vi "play_AFM_PI.vi"() -> ()   [LabVIEW 2017]
uses:
  controls/controlParams_tracktraj.ctl
  <vilib>/Analysis/Matrix/Datatypes/RealMatrix.ctl
  fpga_fp_interface_lib/fpga_interface_types/boolean_indicators.ctl
  <vilib>/userdefined/High Color/nirio_resource_hc.ctl
  <vilib>/Utility/error.llb/DialogType.ctl
  <vilib>/Utility/file.llb/Read From Spreadsheet File (DBL).vi
  <vilib>/FPGAPlugInAG/cRIO-9082/niLvFpga_Open_cRIO-9082.vi
  <vilib>/rvi/interface/common/dynamic/niFpgaDynamicAddResources.vi
  <vilib>/FPGAPlugInAG/Dynamic/niLvFpga_Reset_Dynamic.vi
  <vilib>/rvi/interface/common/niFpgaWaitOnOcc.vi
  <vilib>/Utility/error.llb/Error Cluster From Error Code.vi
  <vilib>/rvi/errors/niLvFpgaAdjustHostInterfaceError.vi
  <vilib>/FPGAPlugInAG/Dynamic/niLvFpga_Run_Dynamic.vi
  fpga_fp_interface_lib/write_FP_data_to_fpga.vi
  fpga_fp_interface_lib/acquire_fp_yk_FIFO.vi
  <vilib>/Utility/file.llb/Write To Spreadsheet File (DBL).vi
  <vilib>/Analysis/Matrix/Numeric/Conversions/Array To Matrix - RA2.vi
  <vilib>/FPGAPlugInAG/Dynamic/niLvFpga_Close_Dynamic.vi
  <vilib>/rvi/interface/nirviOpenFPGA/nirviOpenFPGA.xnode
  FPGA Bitfiles/XYpeizocontrol_FPGATargetSPARTA_AFM_PI_control.lvbitx
  <vilib>/rvi/interface/nirviMethod/nirviMethod.xnode
  <vilib>/rvi/interface/nirviReadWriteControl/nirviReadWriteControl.xnode
  <vilib>/rvi/interface/nirviCloseFPGA/nirviCloseFPGA.xnode
  <vilib>/FPGAPlugInAG/Dynamic/niLvFpga_ConfigureFifo_Dynamic.vi
  <vilib>/rvi/errors/niLvFpgaMergeErrorWithErrorCode.vi
  <vilib>/rvi/interface/Simulation/niFpgaSimulationCallBeginRW.vi
  <vilib>/Analysis/Matrix/NI_Matrix.lvlib
  <vilib>/FPGAPlugInAG/Dynamic/niLvFpga_WriteFifo_Dynamic.vi
  NiFpgaLv.dll
panel:
  in  "Tab Control":enum32{"MAIN", "Page 1", "Debug Info"}(tab)
  out "XY Graph":cluster{dbl[], "2D Data Out":dbl[]}[](graph)
  in  "traj_path":path=path "Z:/mpc-journal/step-exps/ref_traj_track.csv"
  in  "TsTicks":i32=1600
  in  "umax":dbl=1.0 format="%#_13g"
  in  "ymax":dbl=4.0 format="%#_13g"
  in  "Iters":i32=25
  in  "SettleTicks":i32=10
  in  "outputDataPath":path=path "Z:/mpc-journal/step-exps/expOut_multiAxis_tmp.csv"
  in  "Kp":sgl
  in  "Ki":dbl=0.125346917944 format="%#_13g"
  in  "ABORT":bool
  out "result_data":T1
  out "boolean  indicators":T2
  out "u_k out":fxp<+/-,32,5>
  out "size(s) 2":i32[](array[numeric])
  out "error out":errorcluster
  out "Actual Depth":u32
  out "error out 2":errorcluster
  out "elements left":i32=1
  in  "Cluster":T3={"umax"=3.0, "y_ref(k)"=0.0, "Ki"=0.0, "y(k) (from plant)"=0.0, "ND"=0, "NS"=0, "u_Kx_ref(k)"=0.0, "du_max"=3.0, "NS_obs"=0, "NS_control"=0, "Kp"=0.0} {"Kp" format="%#_13g"; "du_max" format="%#_13g"; "u_Kx_ref(k)" format="%#_13g"; "Ki" format="%#_13g"; "y_ref(k)" format="%#_13g"; "umax" format="%#_13g"}
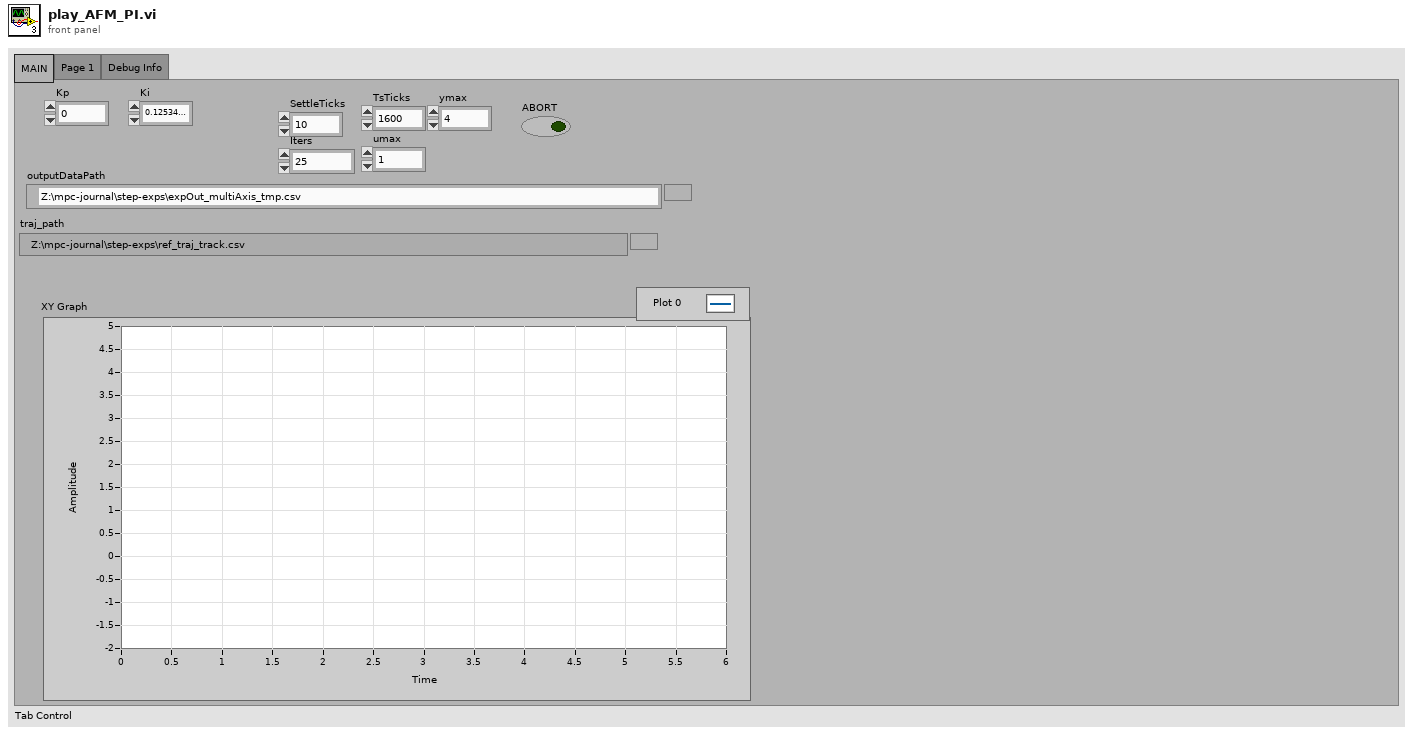
[diagram p1: front panel]
types:
  T1 = typedef "NI_Matrix.lvlib/RealMatrix.ctl" = dbl[][]
  T2 = typedef "boolean_indicators.ctl" = cluster{"unstable-z-traj":bool, "input fifo time-out":bool, "logging fifo timeout":bool, "scanning finished":bool, "unstable-x-traj":bool, "unstable-y-traj":bool, "ABORT":bool, "All Measurements Done":bool, "fpga_finished":bool}
  T3 = typedef "controlParams_tracktraj.ctl" = cluster{"umax":sgl, "y_ref(k)":sgl, "Ki":sgl, "y(k) (from plant)":sgl, "ND":i16, "NS":i16, "u_Kx_ref(k)":sgl, "du_max":sgl, "NS_obs":i16, "NS_control":i16, "Kp":sgl}
  T4 = typedef "nirio_resource_hc.ctl" = tag
  T5 = cluster{"unstable-z-traj":bool, "input fifo time-out":bool, "logging fifo timeout":bool, "scanning finished":bool, "unstable-x-traj":bool, "unstable-y-traj":bool, "ABORT":bool, "All Measurements Done":bool, "fpga_finished":bool}
  T6 = typedef "DialogType.ctl" = u16
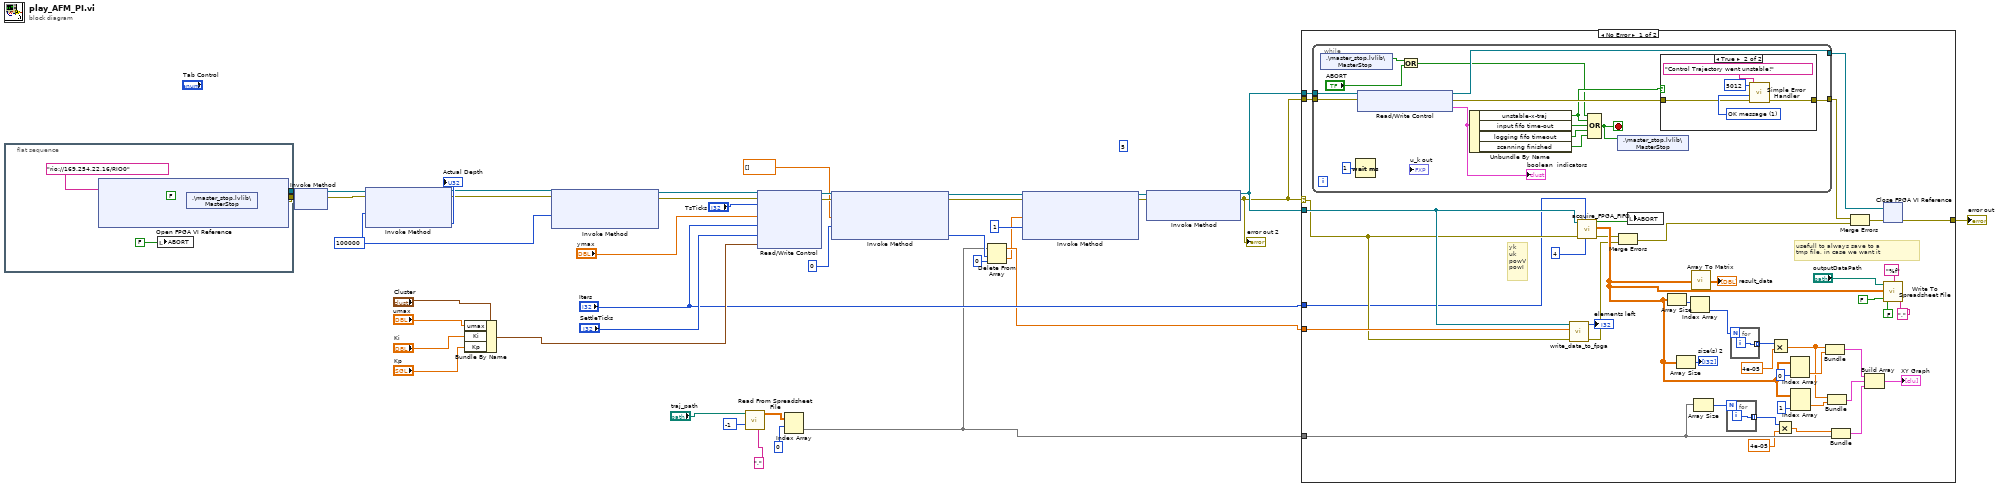
[diagram p0: block diagram]
diagram:
  (unwired) 5
  w34 = 100000
  n1 = flat-sequence {
    tunnel: [w47] -> w33
    tunnel: [w45] -> w4
    frame #0 {
      n2 = xnode "Open FPGA VI Reference"("resource name"=T4 "rio://169.254.22.16/RIO0") -> ("FPGA VI Reference Out"=w47:refnum<k20>, "error out"=w44:errorcluster)  [unwired: 1 in]
      n3 = local write "ABORT"(FALSE ("MasterStop")) -> ()
      n4 = shared-variable ".\\master_stop.lvlib\\MasterStop"(FALSE ("MasterStop"), error in=w44) -> (error out=w45:errorcluster)
    }
  }
  n5 = xnode "Invoke Method"("FPGA VI Reference In"=w33, "error in"=w4) -> ("FPGA VI Reference Out"=w39:refnum<k20>, "error out"=w38:errorcluster)
  n6 = xnode "Invoke Method"("FPGA VI Reference In"=w39, "error in"=w38, "Requested Depth"=w34) -> ("FPGA VI Reference Out"=w7:refnum<k20>, "error out"=w6:errorcluster, "Actual Depth"=→"Actual Depth":u32)
  n7 = Bundle By Name(cluster="Cluster", "umax"="umax", "Ki"="Ki", "Kp"="Kp") -> (w24:T3)
  n8 = xnode "Invoke Method"("FPGA VI Reference In"=w7, "error in"=w6, "Requested Depth"=w34) -> ("FPGA VI Reference Out"=w36:refnum<k20>, "error out"=w35:errorcluster)  [unwired: 1 out]
  n9 = call-poly <vilib>:"Read From Spreadsheet File.vi"("delimiter (\\t)"=",", "number of rows (all:-1)"=-1, "file path (dialog if empty)"="traj_path") -> ("all rows"=w28:dbl[][])  [unwired: 4 in, 4 out]
  n10 = xnode "Read/Write Control"("FPGA VI Reference In"=w36, "error in"=w35, "TsTicks"="TsTicks", "ymax"="ymax", "iters"="Iters", "Settle Ticks"="SettleTicks", "ControlParms"=w24) -> ("FPGA VI Reference Out"=w20:refnum<k20>, "error out"=w19:errorcluster)
  n11 = Index Array(array=w28, index (row)=0 ("dimension size")) -> (element=w1:dbl[])  [unwired: 1 in]
  n12 = xnode "Invoke Method"("FPGA VI Reference In"=w20, "error in"=w19, "Data"=sgl[] [], "Timeout (ms)"=0 ("index")) -> ("FPGA VI Reference Out"=w16:refnum<k20>, "error out"=w15:errorcluster, "Empty Elements Remaining"=w13:u32)
  n13 = Delete From Array(array=w1, length=w13, index=0) -> (deleted portion=w2:dbl[], array with subset deleted=w11:dbl[])
  n14 = xnode "Invoke Method"("FPGA VI Reference In"=w16, "error in"=w15, "Data"=w2, "Timeout (ms)"=1) -> ("FPGA VI Reference Out"=w18:refnum<k20>, "error out"=w17:errorcluster)  [unwired: 1 out]
  n15 = xnode "Invoke Method"("FPGA VI Reference In"=w18, "error in"=w17) -> ("FPGA VI Reference Out"=w22:refnum<k20>, "error out"=w5:errorcluster)  [unwired: 1 in]
  "error out 2" <- w5
  n16 = case shown="No Error" w5 {
    selector: w5 -> [w64 w113]
    tunnel: [w55 w113] -> w10
    tunnel: w22 -> [w88 _]
    tunnel: w5 -> [w87 _]
    tunnel: "Iters" -> [w56 _]
    tunnel: w22 -> [w66 _]
    tunnel: w11 -> [w65 _]
    tunnel: w1 -> [w52 _]
    frame No Error {
      # "yk\nuk\npowV\npowI"
      # "usefull to always save to a \ntmp file, in case we want it"
      n17 = while {
        tunnel: w88 -> [w105]
        tunnel: w87 -> [w104]
        tunnel: [w102] -> w86
        tunnel: [w101] -> w85
        stop <- w100 stop-if-true
        n18 = shared-variable ".\\master_stop.lvlib\\MasterStop"() -> (w95:bool)  [unwired: 1 in, 1 out]
        n19 = Wait (ms)(milliseconds to wait=u32 1) -> ()  [unwired: 1 out]
        n20 = xnode "Read/Write Control"("FPGA VI Reference In"=w105, "error in"=w104) -> ("FPGA VI Reference Out"=w101:refnum<k20>, "error out"=w103:errorcluster, "boolean  indicators"=w99:T5)
        "boolean  indicators" <- w99
        n21 = Or(x=w95, y="ABORT") -> (x .or. y?=w93:bool)
        n22 = Unbundle By Name(w99) -> ("unstable-x-traj"=w97:bool, "input fifo time-out"=w98:bool, "logging fifo timeout"=w96:bool, "scanning finished"=w92:bool)
        n23 = Compound Arithmetic op=OR(w93, w97, w98, w96, w92) -> (w100:bool)
        n24 = shared-variable ".\\master_stop.lvlib\\MasterStop"(w100) -> ()  [unwired: 1 in, 1 out]
        n25 = case shown="True" w97 {
          tunnel: w103 -> [w107 w109]
          tunnel: [w107 w108] -> w102
          frame False {
          }
          frame True {
            w112 = T6 1 items=["no dialog", "OK message", "continue or stop message", "OK message + warnings", "continue/stop + warnings"] ("type of dialog (OK msg:1)")
            n26 = call <vilib>:"Simple Error Handler.vi"("error code (no error:0)"=5012, "error source (\" \")"="Control Trajectory went unstable!" ("error source (\" \")"), "type of dialog (OK msg:1)"=w112, "error in (no error)"=w109) -> ("error out"=w108:errorcluster)  [unwired: 1 in, 4 out]
          }
        }
      }
      n27 = call-poly "write_data_to_fpga.vi"("error in"=w64, "all rows"=w65, "FPGA Interface"=w66) -> ("error out"=w61:errorcluster, "elements left"=→"elements left":i32)  [unwired: 7 in]
      n28 = call-poly "acquire_FPGA_FIFO.vi"("numChannels"=u8 4 ("y"), "Iters"=w56, "error in (no error)"=w64, "FPGA Interface"=w66) -> ("error out"=w63:errorcluster, "2D Data Out"=w82:dbl[][], "acquisition done"=w84:bool)  [unwired: 3 in, 2 out]
      n29 = Merge Errors(w63, w61) -> (w62:errorcluster)
      n30 = local write "ABORT"(w84) -> ()
      n31 = Array Size(array=w82) -> (size(s)=w76:i32[])
      n32 = Array Size(array=w82) -> (size(s)=→"size(s) 2":i32[])
      n33 = Index Array(array=w76) -> (element=w75:i32)  [unwired: 1 in]
      n34 = call-poly <vilib>:"Array To Matrix.vi"("Real 2D Array"=w82) -> ("Real Matrix"=→"result_data":T1)
      n35 = Array Size(array=w52) -> (size(s)=w51:i32)
      n36 = for {
        N: w51 -> [_]
        tunnel: [w90] -> w49 mode=indexing
        i -> [w90]
      }
      n37 = for {
        N: w75 -> [_]
        tunnel: [w91] -> w74 mode=indexing
        i -> [w91]
      }
      n38 = Multiply(x=w74, y=4e-05) -> (x*y=w59:dbl[])
      n39 = Multiply(x=w49, y=4e-05) -> (x*y=w48:dbl[])
      n40 = Index Array(array=w82, index (col)=0 ("disabled index (col)")) -> (element=w72:dbl[])  [unwired: 1 in]
      n41 = Index Array(array=w82, index (col)=1 ("index (row)")) -> (element=w71:dbl[])  [unwired: 1 in]
      n42 = Bundle(w59, "2D Data Out"=w72) -> (w53:cluster{dbl[], "2D Data Out":dbl[]})  [unwired: 1 in]
      n43 = Bundle(w59, "2D Data Out"=w71) -> (w54:cluster{dbl[], "2D Data Out":dbl[]})  [unwired: 1 in]
      n44 = Bundle(w48, "all rows"=w52) -> (w58:cluster{dbl[], "all rows":dbl[]})  [unwired: 1 in]
      n45 = Merge Errors(w86, w62) -> (w89:errorcluster)
      n46 = Build Array(w53, w54, w58) -> (→"XY Graph":cluster{dbl[], "all rows":dbl[]}[])
      n47 = xnode "Close FPGA VI Reference"("FPGA VI Reference In"=w85, "error in"=w89) -> ("error out"=w55:errorcluster)
      n48 = call-poly <vilib>:"Write To Spreadsheet File.vi"("delimiter (\\t)"=",", "transpose? (no:F)"=FALSE, "format (%.3f)"="%f", "append to file? (new file:F)"=FALSE, "2D data"=w82, "file path (dialog if empty)"="outputDataPath") -> ()  [unwired: 2 in, 1 out]
    }
    frame Error {
    }
  }
  "error out" <- w10
